vi "get_rumble_video_metadata.vi"(0 "HTTP client handle":T3, 1 "Keyword ignore case (T)":bool=TRUE, 2 "Keyword":string, 5 "Video ID":i32, 11 "error in (no error)":errorcluster) -> (3 "Keyword found":bool, 4 "client handle out":T3, 6 "Video metadata":T2, 8 "Query result":T1, 15 "error out":errorcluster)   [LabVIEW 2023]
uses:
  <vilib>/httpClient/ClientHandle.ctl
  bce9b43a-9ec8-432c-8d9a-e85697075c85.vi
  a7c33b3b-108a-4440-982b-1fe2c4f3b8f3.vi
  <vilib>/Utility/error.llb/Trim Whitespace One-Sided.vi
  <vilib>/JDP Science/JSONtext/JSON text to Variant.vi
  <vilib>/JDP Science/JSONtext/LVClass Serializer/JSONtext LVClass Serializer.lvclass
  <vilib>/regexp/Match Regular Expression.xnode
  <vilib>/httpClient/LabVIEWHTTPClient.lvlib
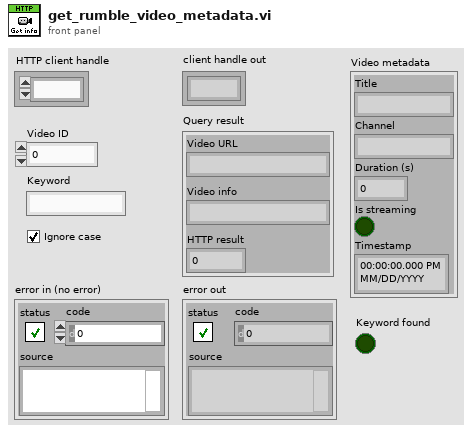
[diagram p1: front panel]
types:
  T1 = cluster{"Video URL":string, "Video info":string, "HTTP result":i32}
  T2 = cluster{"Title":string, "Channel":string, "Duration (s)":i32, "Is streaming":bool, "Timestamp":timestamp}
  T3 = typedef "LabVIEWHTTPClient.lvlib/ClientHandle.ctl" = refnum<k1>
  T4 = cluster{"fractional second":dbl, "second":i32, "minute":i32, "hour":i32, "day of month":i32, "month":i32, "year":i32, "day of week":i32, "day of year":i32, "DST":i32}
  T5 = cluster{"title":string, "author_name":string, "duration":i32, "html":string}
  T6 = cluster{"title":string, "author_name":string, "duration":i32, bool, "time stamp":timestamp}
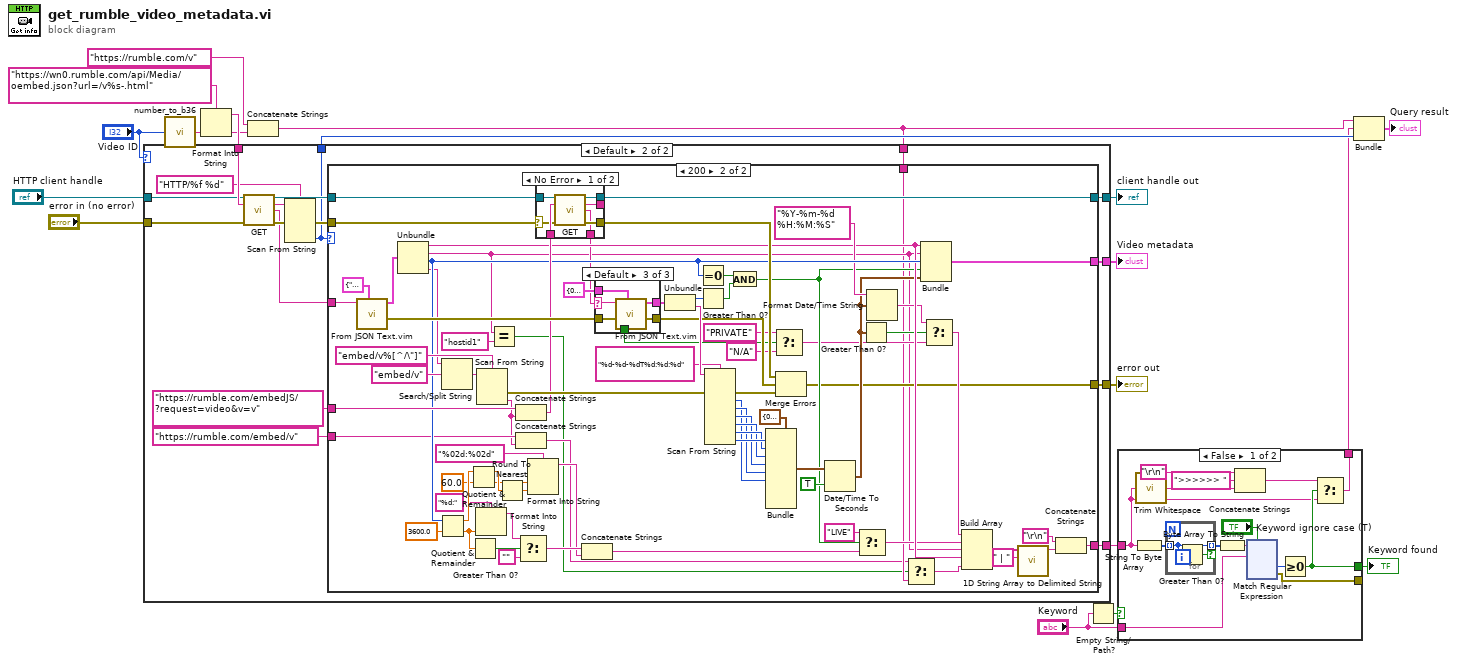
[diagram p0: block diagram]
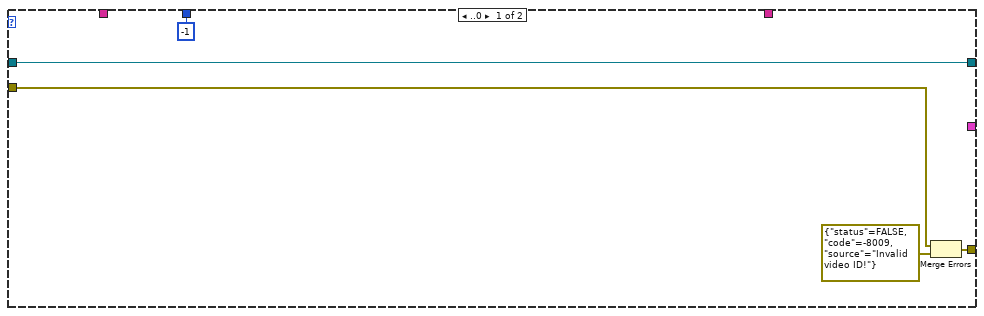
[diagram p3: hidden frame]
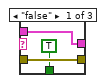
[diagram p5: hidden frame]
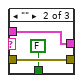
[diagram p6: hidden frame]
diagram:
  n1 = call "number_to_b36.vi"("Number"="Video ID") -> ("Base36 string"=w10:string)
  n2 = Format Into String(format string="https://wn0.rumble.com/api/Media/oembed.json?url=/v%s-.html", w10) -> (resulting string=w17:string)  [unwired: 2 in, 1 out]
  n3 = Concatenate Strings("https://rumble.com/v", w10) -> (w7:string)
  n4 = case shown="Default" "Video ID" {
    tunnel: w17 -> [_ w40]
    tunnel: [w23 w33] -> w16
    tunnel: "HTTP client handle" -> [w23 w39]
    tunnel: "error in (no error)" -> [w21 w38]
    tunnel: [_ w37] -> w13
    tunnel: [w19 w30] -> w12
    tunnel: w7 -> [_ w29]
    tunnel: [_ w31] -> w2
    tunnel: [-1 w27] -> w8
    frame ..0 {
      n5 = Merge Errors(w21, errorcluster {"status"=FALSE, "code"=-8009, "source"="Invalid video ID!"} ("error in (no error)")) -> (w19:errorcluster)
    }
    frame Default {
      n6 = call <vilib>:"GET.vi"("client handle"=w39, "url"=w40, "error in (no error)"=w38) -> ("client handle out"=w34:T3, "headers"=w32:string, "body"=w28:string, "error out"=w36:errorcluster)  [unwired: 9 in]
      n7 = Scan From String(format string="HTTP/%f %d", input string=w32, error in=w36) -> (error out=w35:errorcluster, output 2=w27:i32)  [unwired: 4 in, 2 out]
      n8 = case shown="200" w27 {
        tunnel: [_ w98] -> w37
        tunnel: w35 -> [w42 w93]
        tunnel: w34 -> [w41 w92]
        tunnel: [w41 w91] -> w33
        tunnel: "https://rumble.com/embedJS/?request=video&v=v" -> [_ w75]
        tunnel: [_ w52] -> w31
        tunnel: [w42 w60] -> w30
        tunnel: w29 -> [_ w46]
        tunnel: w28 -> [_ w54]
        tunnel: "https://rumble.com/embed/v" -> [_ w48]
        frame 0, Default {
        }
        frame 200 {
          n9 = call "From JSON Text.vim"("Data Type and Default Value"=T5 {"title"="", "author_name"="", "duration"=0, "html"=""}, "JSON"=w54) -> ("error out"=w99:errorcluster, "Data out"=w117:T5)  [unwired: 8 in]
          n10 = Unbundle(w117) -> ("title"=w72:string, "author_name"=w50:string, "duration"=w74:i32, "html"=w53:string)
          n11 = Quotient & Remainder(x=w74, y=3600.0) -> (x-y*floor(x/y)=w88:dbl, floor(x/y)=w77:dbl)
          n12 = Search/Split String(string=w53, search string/char (-)="embed/v" ("String")) -> (match + rest of string=w119:string)  [unwired: 1 in, 2 out]
          n13 = Quotient & Remainder(x=w88, y=60.0) -> (x-y*floor(x/y)=w86:dbl, floor(x/y)=w81:dbl)
          n14 = Greater Than 0?(x=w77) -> (x > 0?=w85:bool)
          n15 = Format Into String(format string="%d:", w77) -> (resulting string=w76:string)  [unwired: 2 in, 1 out]
          n16 = Scan From String(format string="embed/v%[^/\"]" ("String"), input string=w119) -> (error out=w95:errorcluster, output 1=w47:string)  [unwired: 3 in, 2 out]
          n17 = Equal?(x=w50, y="hostid1") -> (x = y?=w44:bool)
          n18 = Round To Nearest(number=w86) -> (nearest integer value=w80:dbl)
          n19 = Concatenate Strings(w75, w47) -> (w94:string)
          n20 = Concatenate Strings(w48, w47) -> (w45:string)
          n21 = Select(t=w76, s=w85, f="") -> (s? t:f=w83:string)
          n22 = Format Into String(format string="%02d:%02d", w81, w80) -> (resulting string=w79:string)  [unwired: 2 in, 1 out]
          n23 = case shown="No Error" w93 {
            selector: w93 -> [w134 w139]
            tunnel: [w138 w139] -> w90
            tunnel: w94 -> [w137 _]
            tunnel: [w136 _] -> w59
            tunnel: w92 -> [w135 w140]
            tunnel: [w133 w140] -> w91
            tunnel: [w132 _] -> _
            frame No Error {
              n24 = call <vilib>:"GET.vi"("client handle"=w135, "url"=w137, "error in (no error)"=w134) -> ("client handle out"=w133:T3, "headers"=w132:string, "body"=w136:string, "error out"=w138:errorcluster)  [unwired: 9 in]
            }
            frame Error {
            }
          }
          n25 = Concatenate Strings(w83, w79) -> (w70:string)
          n26 = case shown="Default" w59 {
            selector: w59 -> [_ _ w127]
            tunnel: cluster{"live":i32, "pubDate":string} {"live"=0, "pubDate"="0000-00-00T00:00:00"} -> [w122 w126 w131]
            tunnel: [w122 w126 w130] -> w114
            tunnel: w99 -> [w123 w125 w129]
            tunnel: [w123 w125 w128] -> w97
            tunnel: [TRUE FALSE _] -> w58
            frame "false" {
            }
            frame "" {
            }
            frame Default {
              n27 = call "From JSON Text.vim"("Data Type and Default Value"=w131, "error in (no error)"=w129, "JSON"=w127) -> ("error out"=w128:errorcluster, "Data out"=w130:cluster{"live":i32, "pubDate":string})  [unwired: 7 in]
            }
          }
          n28 = Unbundle(w114) -> ("live"=w109:i32, "pubDate"=w110:string)
          n29 = Equal To 0?(x=w74) -> (x = 0?=w113:bool)
          n30 = Greater Than 0?(x=w109) -> (x > 0?=w112:bool)
          n31 = Scan From String(format string="%d-%d-%dT%d:%d:%d", input string=w110, error in=w95) -> (error out=w96:errorcluster, output 1=w102:i32, output 2=w103:i32, output 3=w104:i32, output 4=w105:i32, output 5=w106:i32, output 6=w107:i32)  [unwired: 7 in, 2 out]
          n32 = And(x=w113, y=w112) -> (x .and. y?=w71:bool)
          n33 = Bundle(cluster=T4 {"fractional second"=0.0, "second"=0, "minute"=0, "hour"=0, "day of month"=0, "month"=0, "year"=0, "day of week"=0, "day of year"=0, "DST"=0} ("date time rec"), "second"=w107, "minute"=w106, "hour"=w105, "day of month"=w104, "month"=w103, "year"=w102) -> (w101:T4)  [unwired: 4 in]
          n34 = Select(t="PRIVATE", s=w58, f="N/A") -> (s? t:f=w55:string)
          n35 = Merge Errors(w90, w97, w96) -> (w60:errorcluster)
          n36 = Date/Time To Seconds(1:TRUE ("is UTC (F)"), 2:w101) -> (0:w63:timestamp)
          n37 = Select(t="LIVE", s=w71, f=w70) -> (s? t:f=w69:string)
          n38 = Greater Than 0?(x=w63) -> (x > 0?=w51:bool)
          n39 = Format Date/Time String(time format string (%c)="%Y-%m-%d %H:%M:%S", seconds (now)=w63) -> (date/time string=w62:string)  [unwired: 1 in]
          n40 = Select(t=w45, s=w44, f=w46) -> (s? t:f=w43:string)
          n41 = Bundle("title"=w72, "author_name"=w50, "duration"=w74, w71, "time stamp"=w63) -> (w98:T6)  [unwired: 1 in]
          n42 = Select(t=w62, s=w51, f=w55) -> (s? t:f=w61:string)
          n43 = Build Array(w61, w69, w50, w72, w43) -> (w66:string[])
          n44 = call <vilib>:"1D String Array to Delimited String.vi"("delimiter"=" | ", "string array"=w66) -> ("delimited string"=w64:string)  [unwired: 9 in]
          n45 = Concatenate Strings("\r\n", w64) -> (w52:string)
        }
      }
    }
  }
  "client handle out" <- w16
  "error out" <- w12
  "Video metadata" <- w13
  n46 = Empty String/Path?(string/path="Keyword") -> (empty?=w3:bool)
  n47 = case shown="False" w3 {
    tunnel: w2 -> [w143 w274]
    tunnel: "Keyword" -> [w151 _]
    tunnel: [w147 _] -> w5
    tunnel: [w145 w274] -> w1
    tunnel: [w144 _] -> _
    frame False {
      n48 = String To Byte Array(string=w143) -> (unsigned byte array=w154:u8[])
      n49 = call <vilib>:"Trim Whitespace.vi"("string"=w143) -> ("trimmed string"=w142:string)  [unwired: 1 in]
      n50 = for {
        tunnel: [w156] -> w153 mode=indexing if=w155
        tunnel: w154 -> [w156] mode=indexing
        n51 = Greater Than 0?(x=w156) -> (x > 0?=w155:bool)
      }
      n52 = Byte Array To String(unsigned byte array=w153) -> (string=w152:string)
      n53 = Concatenate Strings("\r\n", ">>>>>> " ("string"), w142) -> (w146:string)
      n54 = xnode "Match Regular Expression"("input string"=w152, "regular expression"=w151, "ignore case? (F)"="Keyword ignore case (T)") -> ("offset past match"=w149:i32, "error out"=w144:errorcluster)  [unwired: 3 in, 3 out]
      n55 = Greater Or Equal To 0?(x=w149) -> (x >= 0?=w147:bool)
      n56 = Select(t=w146, s=w147, f=w143) -> (s? t:f=w145:string)
    }
    frame True {
    }
  }
  "Keyword found" <- w5
  n57 = Bundle(w7, w1, w8) -> (→"Query result":cluster{string, string, i32})  [unwired: 1 in]
